vi "Main.vi"() -> ()   [LabVIEW 2018]
doc: "The myRIO Project template acquires acceleration data from the onboard accelerometer and displays the changes of acceleration values in a waveform chart."
uses:
  <vilib>/FPGAPlugInAG/myRIO-1900/niLvFpga_Open_myRIO-1900.vi
  <vilib>/rvi/interface/common/dynamic/niFpgaDynamicAddResources.vi
  <vilib>/FPGAPlugInAG/Dynamic/niLvFpga_Run_Dynamic.vi
  <vilib>/Utility/error.llb/Error Cluster From Error Code.vi
  <vilib>/rvi/errors/niLvFpgaAdjustHostInterfaceError.vi
  <vilib>/addons/control/pid/pid.llb/PID (DBL).vi
  <vilib>/FPGAPlugInAG/Dynamic/niLvFpga_Close_Dynamic.vi
  <vilib>/rvi/interface/nirviOpenFPGA/nirviOpenFPGA.xnode
  FPGA Bitfiles/Project1_FPGATarget_pulsein_j1g6UUDAEOU.lvbitx
  Sonar myRio/pulse_in.vi
  <vilib>/rvi/interface/nirviMethod/nirviMethod.xnode
  <vilib>/rvi/interface/nirviReadWriteControl/nirviReadWriteControl.xnode
  <vilib>/rvi/interface/nirviCloseFPGA/nirviCloseFPGA.xnode
  <vilib>/rvi/interface/Simulation/niFpgaSimulationCallBeginRW.vi
  NiFpgaLv.dll
  <vilib>/addons/control/pid/NI_PID_pid.lvlib
  <vilib>/ptbypt/NI_PtbyPt.lvlib
panel:
  out "Waveform Graph":dbl[][](graph)
  out "Process Variable and Setpoint":cluster{dbl, dbl}(knob)={0.0, 10.0} scale=0.0..100.0
  out "Manipulated Variable":ext(slide) scale=10.0..20.0
  in  "Output range":cluster{"output high":dbl, "output low":dbl}={"output high"=100.0, "output low"=-100.0} {"output low" format="%.3f"; "output high" format="%.3f"}
  in  "reinitialize? (F)":bool
  in  "PID gains":T1={"proportional gain (Kc)"=1.0, "integral time (Ti, min)"=0.01, "derivative time (Td, min)"=0.0} {"derivative time (Td, min)" format="%.3f"; "integral time (Ti, min)" format="%.3f"; "proportional gain (Kc)" format="%.3f"}
  in  "Setpoint":dbl(knob) scale=10.0..90.0
  in  "Stop":bool
  # "HC-SR04 ultrasonic module to measure distances in the range 2cm – 400cm."
  # "Connection:  Vcc to Pin 1 (Green + Black)   Port A"
  # "Gnd to Pin 12 (Green + Black) Port A"
  # "Trig to Pin 11 (Yellow) Port A"
  # "Echo to Pin 13 (Green) Port A"
  # "PWM to Pin 27 (Purple +Brown) Port A"
  # "Green Needle - PV"
  # "Red Needle - Setpoint"
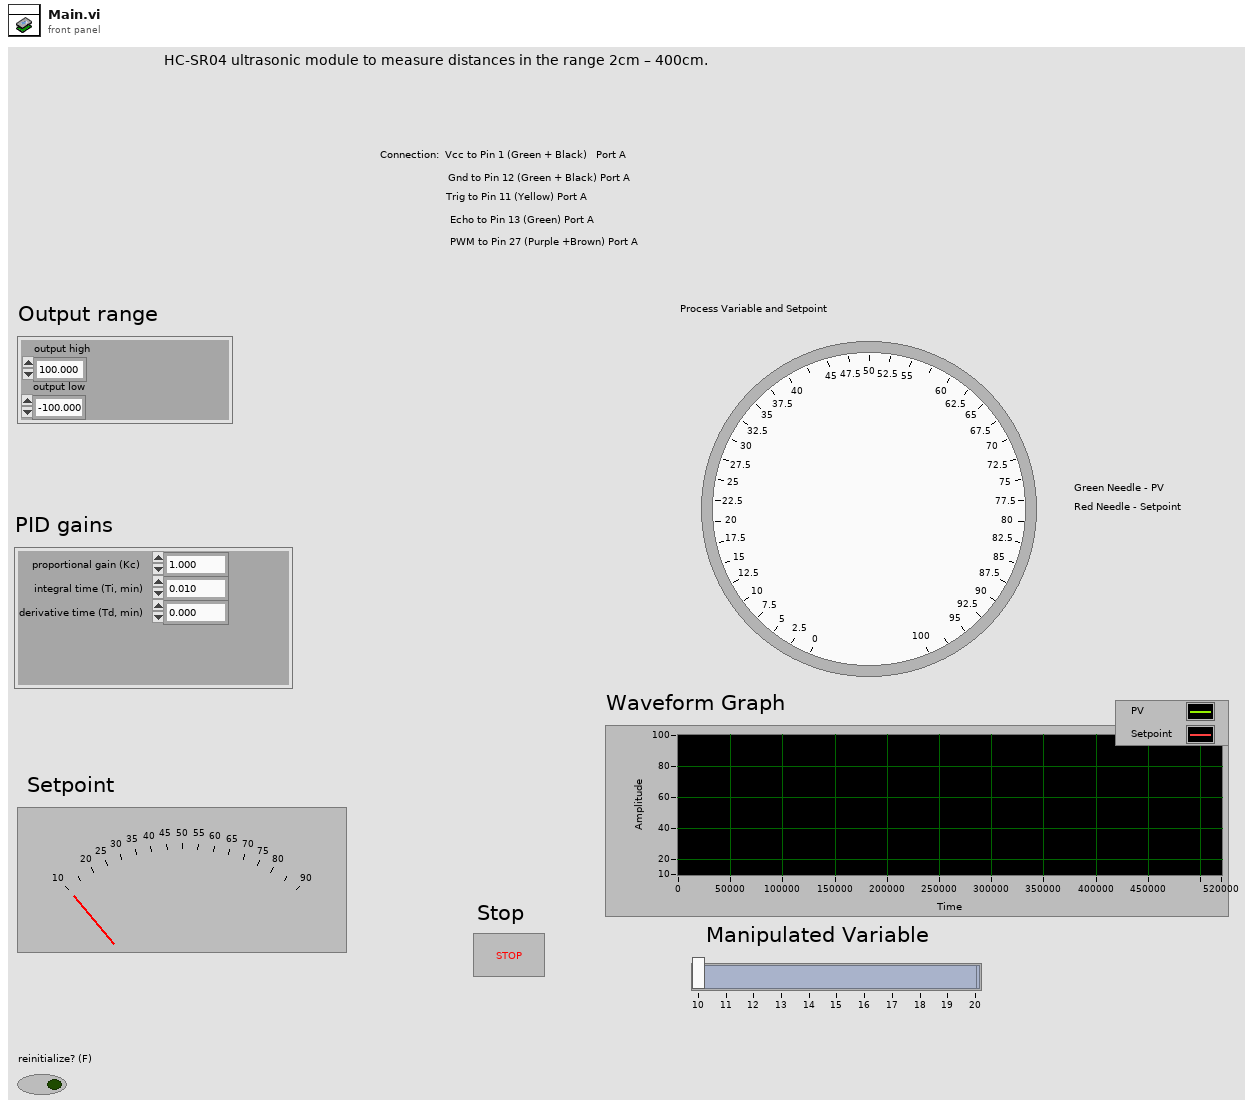
[diagram p1: front panel]
types:
  T1 = cluster{"proportional gain (Kc)":dbl, "integral time (Ti, min)":dbl, "derivative time (Td, min)":dbl}
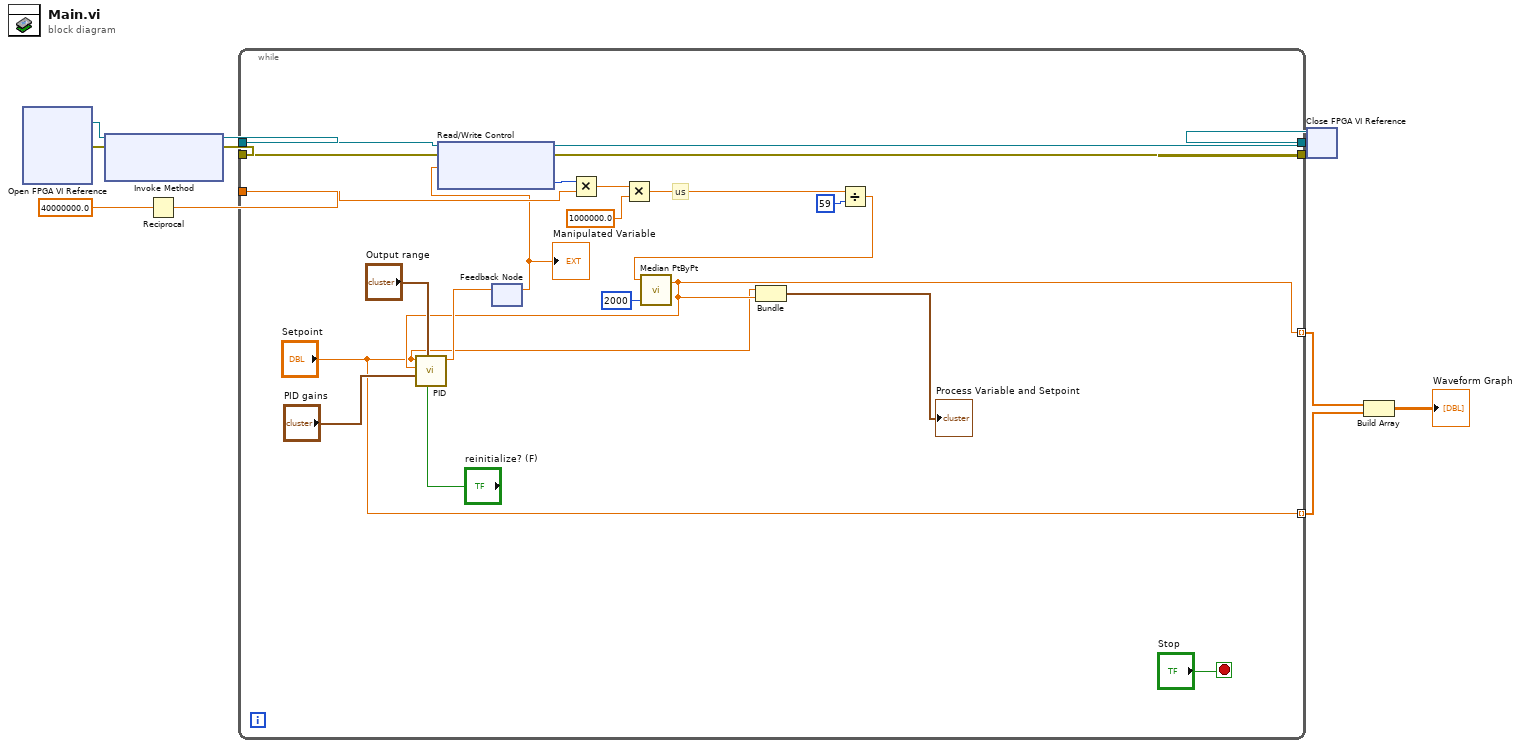
[diagram p0: block diagram]
diagram:
  n1 = xnode "Open FPGA VI Reference"() -> ("FPGA VI Reference Out"=w4:refnum<k20>, "error out"=w5:errorcluster)  [unwired: 2 in]
  n2 = xnode "Invoke Method"("FPGA VI Reference In"=w4, "error in"=w5) -> ("FPGA VI Reference Out"=w6:refnum<k20>, "error out"=w7:errorcluster)  [unwired: 1 in]
  n3 = Reciprocal(x=40000000.0) -> (1/x=w11:dbl)
  n4 = while {
    tunnel: w6 -> [w32]
    tunnel: w7 -> [w31]
    tunnel: [w30] -> w8
    tunnel: [w23] -> w9
    tunnel: w11 -> [w29]
    tunnel: [w13] -> w2 mode=indexing
    tunnel: ["Setpoint"] -> w3 mode=indexing
    stop <- "Stop" stop-if-true
    # "us"
    n5 = feedback #1() -> (w15:dbl)  [unwired: 1 in]
    "Manipulated Variable" <- w15
    n6 = xnode "Read/Write Control"("FPGA VI Reference In"=w32, "error in"=w31, "servo pwm"=w15) -> ("FPGA VI Reference Out"=w30:refnum<k20>, "error out"=w23:errorcluster, "High Period (ticks)"=w27:u32)
    n7 = Multiply(x=w27, y=w29) -> (x*y=w26:dbl)
    n8 = Multiply(x=w26, y=1000000.0) -> (x*y=w24:dbl)
    n9 = Divide(x=w24, y=u32 59) -> (x/y=w18:dbl)
    n10 = call <vilib>:"Median PtByPt.vi"("sample length"=2000, "x"=w18) -> ("median"=w13:dbl)  [unwired: 2 in, 1 out]
    n11 = call-poly <vilib>:"PID.vi"("reinitialize? (F)"="reinitialize? (F)", "output range"="Output range", "PID gains"="PID gains", "process variable"=w13, "setpoint"="Setpoint") -> ("output"=w16:dbl)  [unwired: 5 in, 1 out]
    n12 = feedback-in #1(w16) -> ()
    n13 = Bundle("Setpoint"="Setpoint", "median"=w13) -> (→"Process Variable and Setpoint":cluster{"Setpoint":dbl, "median":dbl})  [unwired: 1 in]
  }
  n14 = xnode "Close FPGA VI Reference"("FPGA VI Reference In"=w8, "error in"=w9) -> ()  [unwired: 1 out]
  n15 = Build Array(w2, w3) -> (→"Waveform Graph":dbl[][])
